vi "save_to_file.vi"   [LabVIEW 2016]
uses:
  <vilib>/Utility/file.llb/Write Delimited Spreadsheet (DBL).vi
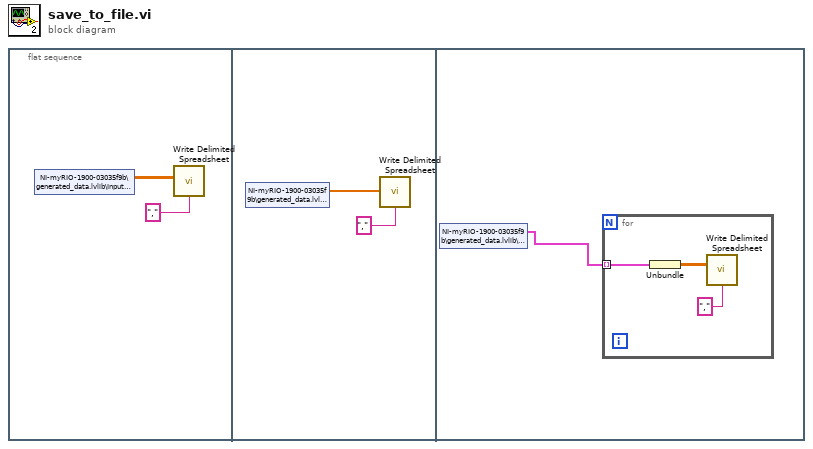
[diagram p0: block diagram]
diagram:
  n1 = flat-sequence {
    frame #0 {
      n2 = shared-variable "NI-myRIO-1900-03035f9b\\generated_data.lvlib\\Input Data"() -> (w1:dbl[][])  [unwired: 1 in, 1 out]
      n3 = call-poly <vilib>:"Write Delimited Spreadsheet.vi"("2D data"=w1, "delimiter (\\t)"=",") -> ()  [unwired: 12 in, 2 out]
    }
    frame #1 {
      n4 = shared-variable "NI-myRIO-1900-03035f9b\\generated_data.lvlib\\Targets"() -> (w4:dbl[])  [unwired: 1 in, 1 out]
      n5 = call-poly <vilib>:"Write Delimited Spreadsheet.vi"("1D data"=w4, "delimiter (\\t)"=",") -> ()  [unwired: 12 in, 2 out]
    }
    frame #2 {
      n6 = shared-variable "NI-myRIO-1900-03035f9b\\generated_data.lvlib\\Weights"() -> (w5:cluster{dbl[][]}[])  [unwired: 1 in, 1 out]
      n7 = for {
        tunnel: w5 -> [w8] mode=indexing
        n8 = Unbundle(w8) -> (w7:dbl[][])
        n9 = call-poly <vilib>:"Write Delimited Spreadsheet.vi"("2D data"=w7, "delimiter (\\t)"=",") -> ()  [unwired: 12 in, 2 out]
      }
    }
  }
